vi "Pulses to speed.vi"(1 "Elapsed time (ms)":i32, 2 "Pulses":i32, 3 "Enc. Diameter (mm)":i32, 4 "No. pulses/rev":i32) -> (0 "Speed (m/s)":dbl)   [LabVIEW 2015]
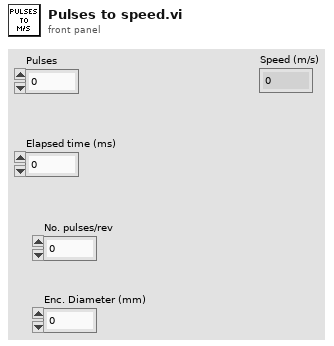
[diagram p1: front panel]
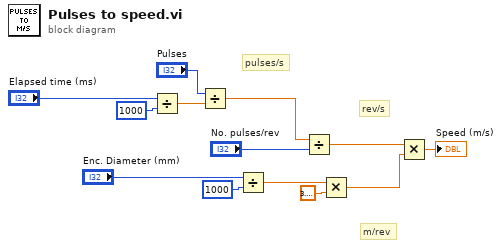
[diagram p0: block diagram]
diagram:
  # "m/rev"
  # "rev/s"
  # "pulses/s"
  n1 = Divide(x="Elapsed time (ms)", y=1000) -> (x/y=w11:dbl)
  n2 = Divide(x="Pulses", y=w11) -> (x/y=w9:dbl)
  n3 = Divide(x="Enc. Diameter (mm)", y=1000) -> (x/y=w1:dbl)
  n4 = Divide(x=w9, y="No. pulses/rev") -> (x/y=w6:dbl)
  n5 = Multiply(x=w1, y=3.141592653589793) -> (x*y=w5:dbl)
  n6 = Multiply(x=w6, y=w5) -> (x*y=→"Speed (m/s)":dbl)
